vi "optionsAcq_channel_smoothing.vi"(6 "readWrite":enum16{"read", "write"}(ring), 7 "smoothing":T1, 8 "error in (no error)":errorcluster, 9 "nrOfPasses":u16, 10 "width":u16, 11 "OSAchannel in":refnum<class "OSAchannel.lvclass">) -> (0 "error out":errorcluster, 1 "nrOfPasses read":u16, 2 "width read":u16, 3 "OSAchannel out":refnum<class "OSAchannel.lvclass">, 4 "FTSLib status":i32, 5 "smoothing read":T1)   [LabVIEW 2010, in "OSAchannel.lvclass"]
uses:
  OSAchannel.lvclass
  _misc/Thorlabs_FTS_misc.llb/interferogram_smoothing.ctl
  OSAchannel.lvclass/OSAchannel.ctl
  _dll/LVLib/FTSLib.lvlib
  OSA.lvclass
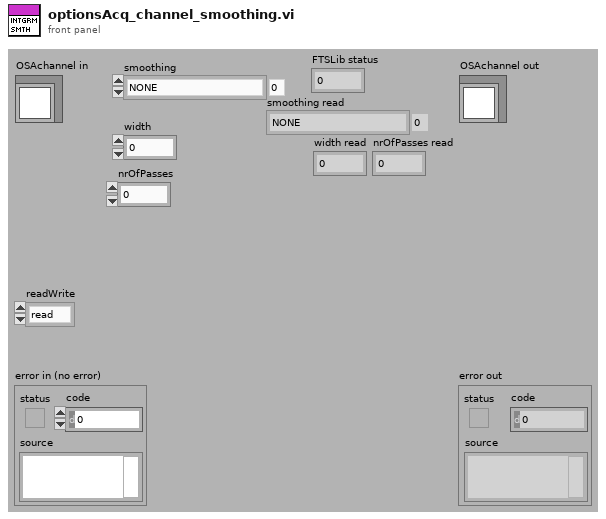
[diagram p1: front panel]
types:
  T1 = typedef "OSA.lvclass/interferogram_smoothing.ctl" = enum16{"NONE", "BINOMIAL", "SAVITSKY_GOLAY", "FOURIER", "MOVING_AVERAGE", "GAUSSIAN"}
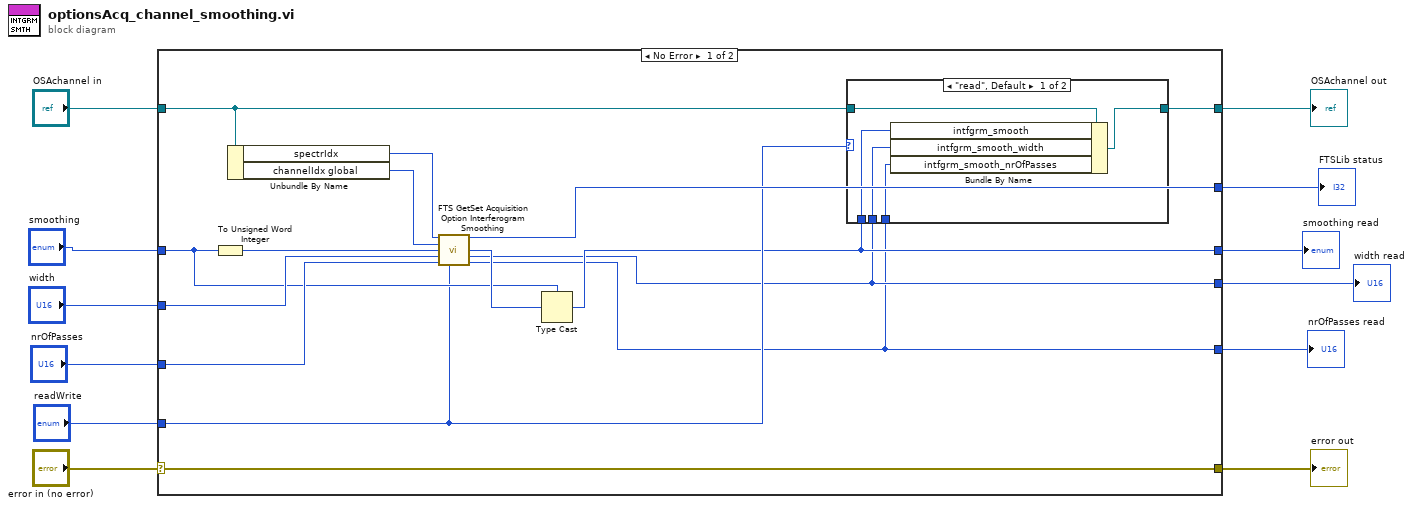
[diagram p0: block diagram]
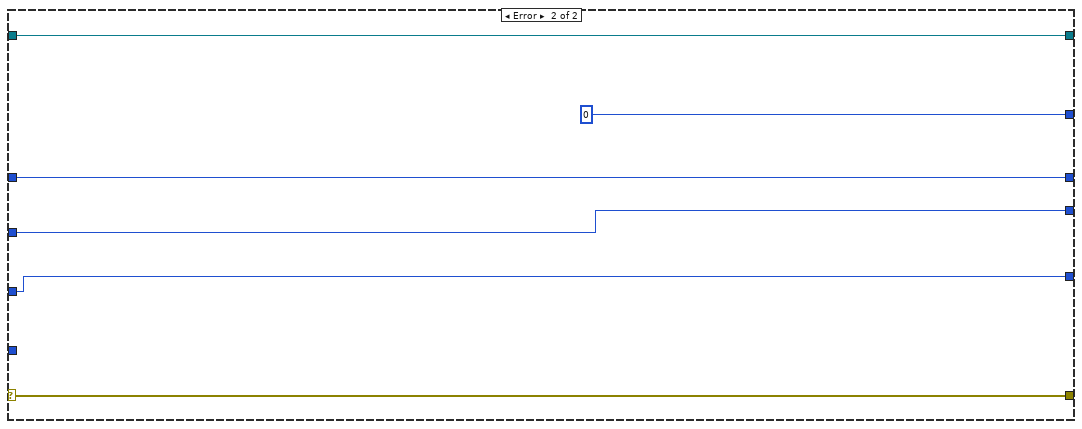
[diagram p3: hidden frame]
diagram:
  n1 = case shown="No Error" "error in (no error)" {
    selector: "error in (no error)" -> [w27 w39]
    tunnel: [w27 w39] -> w11
    tunnel: [w17 w38] -> w9
    tunnel: "OSAchannel in" -> [w18 w38]
    tunnel: "smoothing" -> [w19 w37]
    tunnel: "width" -> [w24 w35]
    tunnel: "nrOfPasses" -> [w23 w34]
    tunnel: "readWrite" -> [w16 _]
    tunnel: [w22 0 ("FTSLib status")] -> w4
    tunnel: [w15 w37] -> w3
    tunnel: [w14 w35] -> w2
    tunnel: [w13 w34] -> w1
    frame No Error {
      n2 = To Unsigned Word Integer(number=w19) -> (unsigned 16bit integer=w21:u16)
      n3 = Unbundle By Name(w18) -> ("spectrIdx"=w26:u16, "channelIdx global"=w25:u16)
      n4 = call "FTS GetSet Acquisition Option Interferogram Smoothing.vi"("spectrIdx"=w26, "channel"=w25, "smoothingType"=w21, "width"=w24, "nrOfPasses"=w23, "readWrite"=w16) -> ("FTSLib status"=w22:i32, "smoothingType read"=w20:u16, "width read"=w14:u16, "nrOfPasses read"=w13:u16)  [unwired: 6 in]
      n5 = Type Cast(type=w19, x=w20) -> (*(type *) &x=w15:T1)
      n6 = case shown="\"read\", Default" w16 {
        tunnel: w18 -> [w32 w33]
        tunnel: [w31 w33] -> w17
        tunnel: w15 -> [w30 _]
        tunnel: w14 -> [w29 _]
        tunnel: w13 -> [w28 _]
        frame "read", Default {
          n7 = Bundle By Name(cluster=w32, "intfgrm_smooth"=w30, "intfgrm_smooth_width"=w29, "intfgrm_smooth_nrOfPasses"=w28) -> (w31:refnum<class "OSAchannel.lvclass">)
        }
        frame "write" {
        }
      }
    }
    frame Error {
    }
  }
  "error out" <- w11
  "OSAchannel out" <- w9
  "FTSLib status" <- w4
  "smoothing read" <- w3
  "width read" <- w2
  "nrOfPasses read" <- w1
